vi "rsmxo_LV2015_Hardcopy_Example.vi"() -> ()   [LabVIEW 2015]
uses:
  <instrlib>/Rohde&Schwarz MXO Oscilloscopes/Rohde&Schwarz MXO Oscilloscopes.lvlib
panel:
  in  "Comment Message":string="My Comment" caption="Message (\"Message\")"
  in  "Instrument File name":string="MyScreenshot.png"
  out "Screenshot":picture
  in  "VISA resource name":refnum<visa-resource-name>="TCPIP::10.112.0.157::hislip0"
  in  "Target PC File":path=path "C:/temp/PC_Screenshot.png"
  in  "Reset":bool
  in  "ID Query":bool=TRUE
  # "Rohde & Schwarz MXO Oscilloscopes Series\nHardcopy Example"
  # "Before running, change the VISA resource name to fit your device:\n- For LAN interface use TCPIP::<IP_Address>::INSTR e.g. TCPIP::10.64.0.178::INSTR\n- For USB interface use USB0::0x0AAD::<PID>::<SN>::INSTR e.g. USB0::0x0AAD::0x01D6::101457::INSTR\n- For GPIB interface use the GPIB::<Address>::INSTR e.g. GPIB::28::INSTR"
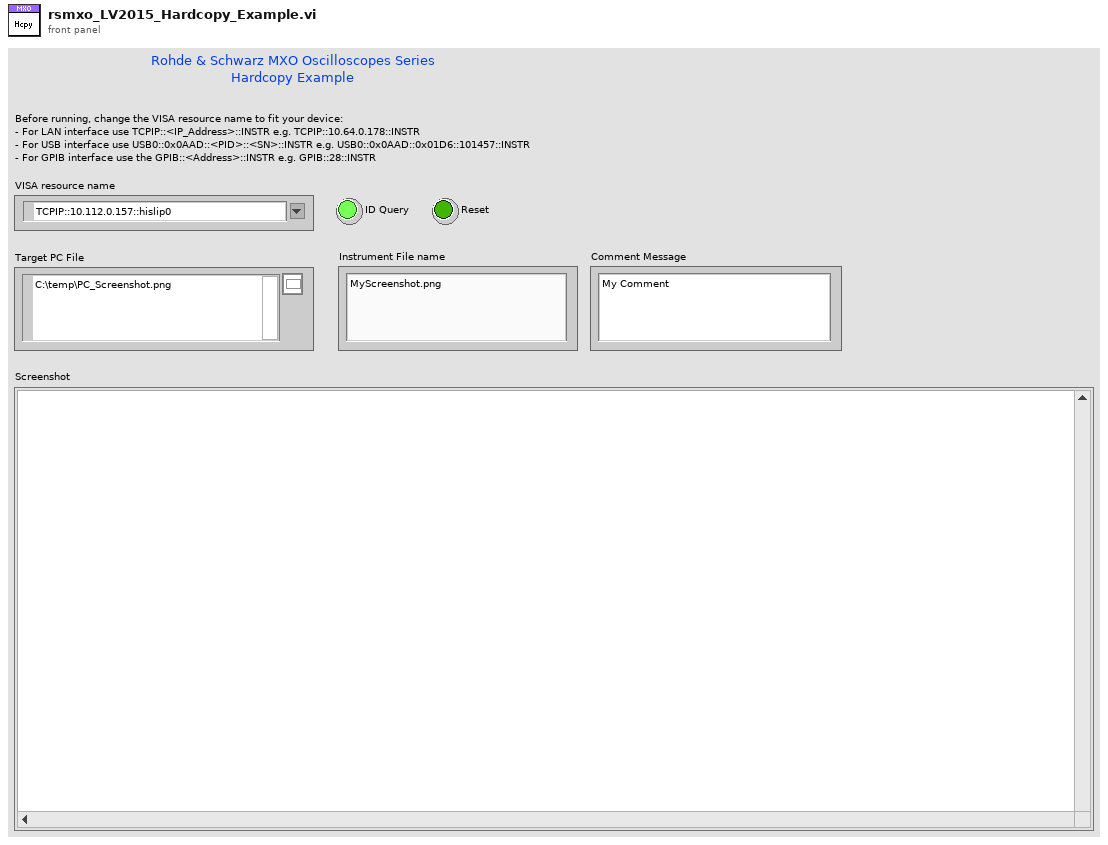
[diagram p1: front panel]
types:
  T1 = typedef "imagedata.ctl" = cluster{"image type":i32, "image depth":i32, "image":u8[], "mask":u8[], "colors":u32[], "Rectangle":cluster{"left":i16, "top":i16, "right":i16, "bottom":i16}}
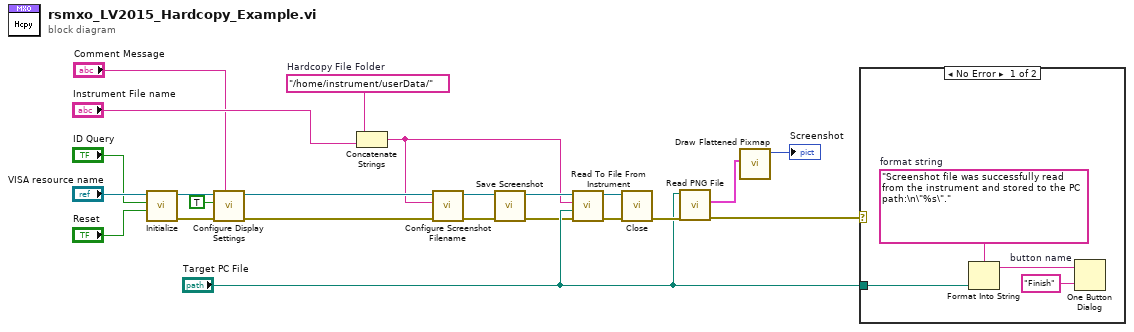
[diagram p0: block diagram]
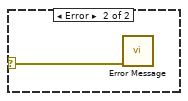
[diagram p2: hidden frame]
diagram:
  w4 = "/home/instrument/userData/"  # Hardcopy File Folder
  n1 = call <instrlib>:"Initialize.vi"("Reset (T: Reset)"="Reset", "ID Query (T: Check)"="ID Query", "VISA resource name"="VISA resource name") -> ("error out"=w11:errorcluster, "VISA resource name out"=w10:refnum<visa-resource-name>)  [unwired: 7 in]
  n2 = call <instrlib>:"Configure Display Settings.vi"("Message (\"Message\")"="Comment Message", "error in (no error)"=w11, "Display Update (Off)"=TRUE, "VISA resource name"=w10) -> ("error out"=w8:errorcluster, "VISA resource name out"=w7:refnum<visa-resource-name>)  [unwired: 6 in]
  n3 = Concatenate Strings(w4, "Instrument File name") -> (w1:string)
  n4 = call <instrlib>:"Configure Screenshot Filename.vi"("error in (no error)"=w8, "Filename (\"filename\")"=w1, "VISA resource name"=w7) -> ("error out"=w6:errorcluster, "VISA resource name out"=w5:refnum<visa-resource-name>)  [unwired: 7 in]
  n5 = call <instrlib>:"Save Screenshot.vi"("error in (no error)"=w6, "VISA resource name"=w5) -> ("error out"=w13:errorcluster, "VISA resource name out"=w12:refnum<visa-resource-name>)  [unwired: 8 in]
  n6 = call <instrlib>:"Read To File From Instrument.vi"("error in (no error)"=w13, "Target PC File"="Target PC File", "Source Instrument File"=w1, "VISA resource name"=w12) -> ("error out"=w22:errorcluster, "VISA resource name out"=w23:refnum<visa-resource-name>)  [unwired: 6 in]
  n7 = call <instrlib>:"Close.vi"("error in (no error)"=w22, "VISA resource name"=w23) -> ("error out"=w17:errorcluster)  [unwired: 9 in]
  n8 = call <vilib>:"Read PNG File.vi"("error in (no error)"=w17, "path to PNG file"="Target PC File") -> ("error out"=w15:errorcluster, "image data"=w18:T1)  [unwired: 7 in, 1 out]
  n9 = call <vilib>:"Draw Flattened Pixmap.vi"("image data"=w18) -> ("new picture"=→"Screenshot":picture)  [unwired: 8 in]
  n10 = case shown="No Error" w15 {
    selector: w15 -> [_ w28]
    tunnel: "Target PC File" -> [w26 _]
    frame No Error {
      w25 = "Finish"  # button name
      w27 = "Screenshot file was successfully read from the instrument and stored to the PC path:\n\"%s\"."  # format string
      n11 = Format Into String(format string=w27, w26) -> (resulting string=w24:string)  [unwired: 2 in, 1 out]
      n12 = One Button Dialog(message=w24, button name ("OK")=w25) -> ()  [unwired: 1 out]
    }
    frame Error {
      n13 = call <instrlib>:"Error Message.vi"("error in (no error)"=w28) -> ()  [unwired: 10 in, 5 out]
    }
  }
